vi "Filter Cluster Tree_2.vi"(7 "Action":T2=enum."Bundler Insert", 9 "Display Items":T1[](array[typedef]), 10 "Filter Str":string, 11 "Tree Ref":refnum<vi>) -> (0 "error out":errorcluster)   [LabVIEW 2023]
uses:
  controls/action enum.ctl
  cluster/Cluster Element Description.ctl
  LabVIEW-common/Controls/Get-Set Enum.ctl
panel:
  out "Filtered Items":T1[](array[typedef])
  in  "C1":T3
  in  "Tree":string[](tree)
  # "DEBUGGARY"
  # "DEBUG"
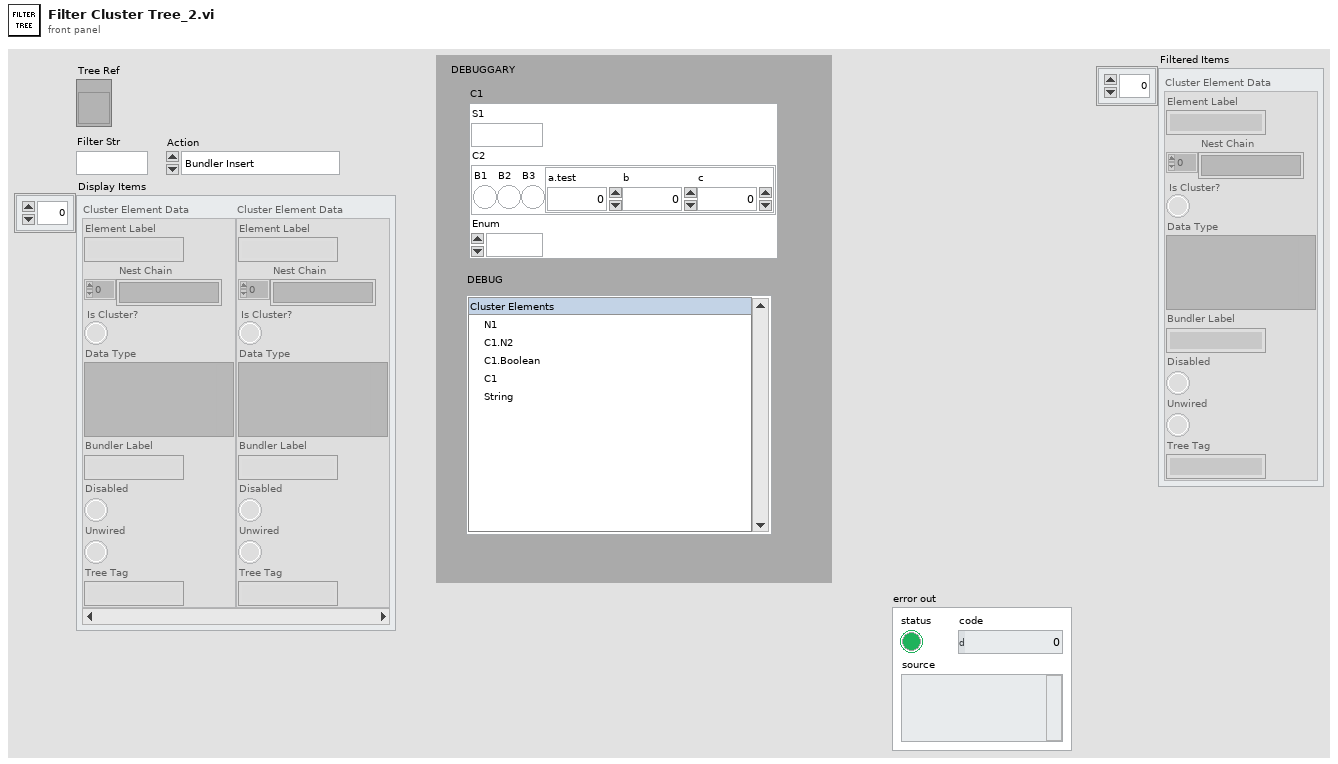
[diagram p1: front panel]
types:
  T1 = typedef "Cluster Element Description.ctl" = cluster{"Element Label":string, "Nest Chain":string[], "Is Cluster?":bool, "Data Type":variant, "Bundler Label":string, "Disabled":bool, "Unwired":bool, "Tree Tag":string}
  T2 = typedef "action enum.ctl" = enum16{"[NONE]", "Wire Bundle", "Wire Unbundle", "Terminal Unbundle", "Terminal Bundle", "Bundler Move Up", "Bundler Move Down", "Bundler Insert", "Bundler Remove", "Bundler Remove Unwired", "Bundler Rearrange", "In Place Insert", "In Place Remove", "In Place Remove Unwired", "In Place Rearrange", "Wire Properties", "Wire Method", "Terminal Properties", "Terminal Method", "Property Move Up", "Property Move Down", "Properties Insert", "Properties Remove", "Properties Remove Unwired", "Properties Rearrange", "Method Change", "Class for Constant", "Class For Control", "Class For Node", "Class Name to Clipboard"}
  T3 = cluster{"S1":string, "C2":cluster{"B1":bool, "B2":bool, "B3":bool, cluster{"a.test":dbl, "b":i32, "c":u8}}, "Enum":enum16{""}}
  T4 = typedef "Get-Set Enum.ctl" = enum16{"Get", "Set"}
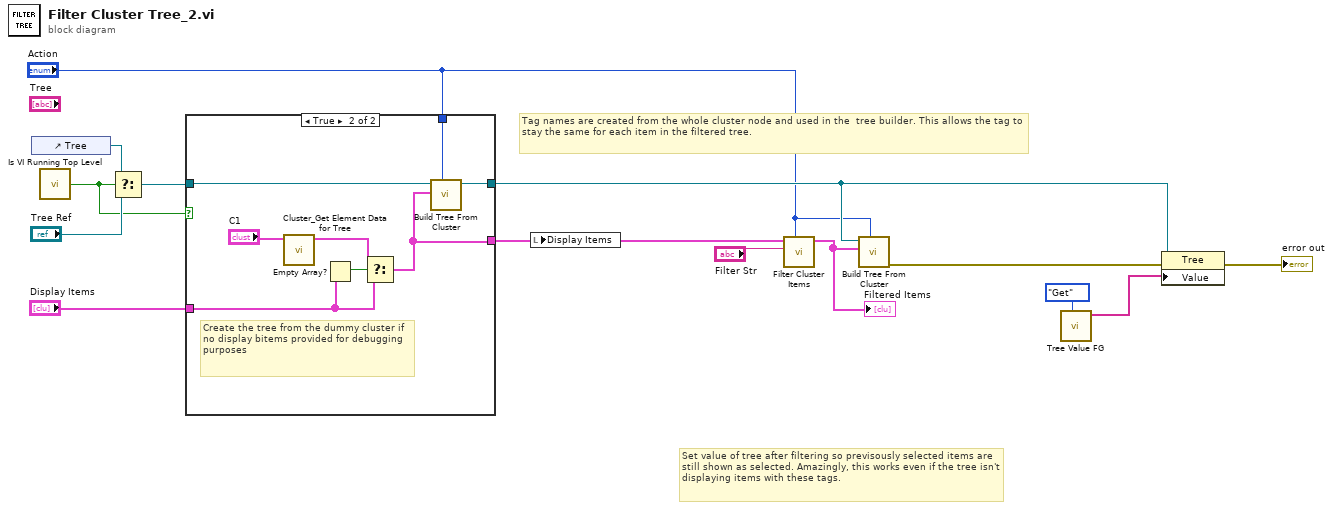
[diagram p0: block diagram]
diagram:
  # "Set value of tree after filtering so previsously selected items are still shown as selected. Amazingly, this works even if the tree isn't displaying items with these tags."
  # "Tag names are created from the whole cluster node and used in the  tree builder. This allows the tag to stay the same for each item in the filtered tree."
  n1 = control-ref of="Tree"() -> (w14:refnum<vi>)
  n2 = call "Is VI Running Top Level.vi"() -> ("Top Level?"=w12:bool)  [unwired: 5 in]
  n3 = Select(t=w14, s=w12, f="Tree Ref") -> (s? t:f=w10:refnum<vi>)
  n4 = case shown="True" w12 {
    tunnel: w10 -> [w16 w24]
    tunnel: [w16 w23] -> w8
    tunnel: [w15 w19] -> w4
    tunnel: "Action" -> [_ w22]
    tunnel: "Display Items" -> [w15 w17]
    frame False {
    }
    frame True {
      # "Create the tree from the dummy cluster if no display bitems provided for debugging purposes"
      n5 = call "Cluster_Get Element Data for Tree.vi"("Data Type"="C1") -> ("Cluster Element Data Aray"=w20:T1[])  [unwired: 10 in]
      n6 = Empty Array?(array=w17) -> (empty?=w18:bool)
      n7 = Select(t=w20, s=w18, f=w17) -> (s? t:f=w19:T1[])
      n8 = call "Build Tree From Cluster.vi"("Action"=w22, "Display Items"=w19, "Tree Ref"=w24) -> ("Tree Ref Out"=w23:refnum<vi>)  [unwired: 7 in, 1 out]
    }
  }
  n9 = local write "Display Items"(w4) -> ()
  n10 = call "Filter Cluster Items.vi"("Action"="Action", "Filter Str"="Filter Str", "Display Items"=w4) -> ("Filtered Items"=w2:T1[])  [unwired: 8 in]
  "Filtered Items" <- w2
  n11 = call "Build Tree From Cluster.vi"("Action"="Action", "Display Items"=w2, "Tree Ref"=w8) -> ("error out"=w6:errorcluster)  [unwired: 7 in, 1 out]
  n12 = call "Tree Value FG.vi"("Get Set Enum"=Get-Set_Enum."Get") -> ("Compiled Value"=w1:string[])  [unwired: 10 in]
  n13 = property class="Tree"(reference=w8, error in=w6, "Value"=w1) -> (error out=→"error out":errorcluster)  [unwired: 1 out]
